vi "Read Constants on Robot.vi"() -> (2 "Constant Names":string[](array[string]), 3 "Constant Values":dbl[](array[numeric]))   [LabVIEW 2013]
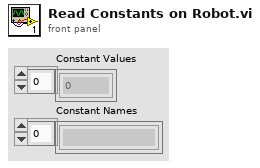
[diagram p1: front panel]
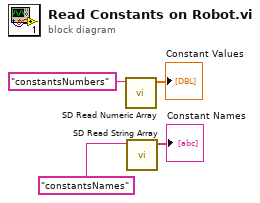
[diagram p0: block diagram]
diagram:
  n1 = call <vilib>:"SD Read Numeric Array.vi"("Name"="constantsNumbers") -> ("Numeric Array"=→"Constant Values":dbl[])  [unwired: 8 in, 2 out]
  n2 = call <vilib>:"SD Read String Array.vi"("Name"="constantsNames") -> ("String Array"=→"Constant Names":string[])  [unwired: 9 in, 1 out]
